vi "Compress with 7Zip.vi"(8 "error in (no error)":errorcluster, 9 "Compressed File Type":string(combo)="7z", 10 "7z File to compress into":path=path "D:/Ab-initio/VASP Calcs/1D_Dislocations/Batch04_20130519/1_DOS.7z", 11 "Folder or file to compress":path=path "D:/Ab-initio/VASP Calcs/1D_Dislocations/Batch04_20130519/1_DOS") -> (0 "error out":errorcluster)   [LabVIEW 2010]
panel:
  out "concatenated string":string="\"C:\\Program Files\\7-Zip\\7za.exe\" a -t7z \"D:\\Ab-initio\\VASP Calcs\\1D_Dislocations\\Batch04_20130519\\1_DOS.7Z\" \"D:\\Ab-initio\\VASP Calcs\\1D_Dislocations\\Batch04_20130519\\1_DOS\""
  in  "7za.exe path":path=path "C:/Program Files/7-Zip/7za.exe"
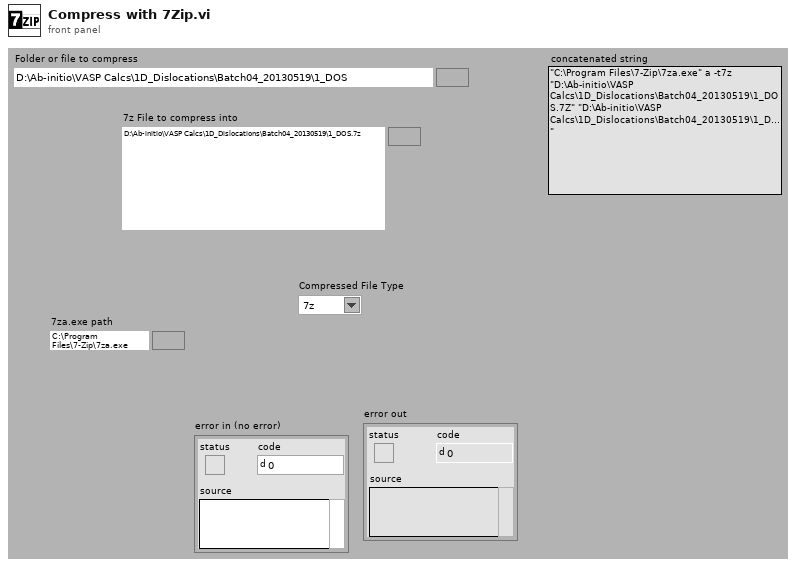
[diagram p1: front panel]
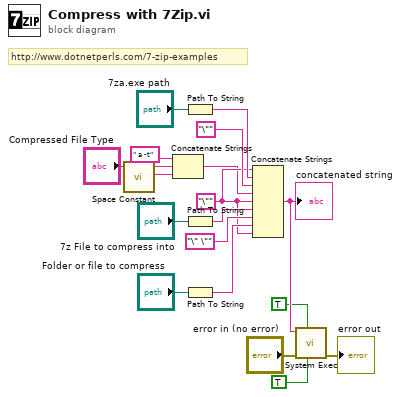
[diagram p0: block diagram]
diagram:
  w11 = "\"" ("string")
  # "http://www.dotnetperls.com/7-zip-examples"
  n1 = call <vilib>:"Space Constant.vi"() -> ("String"=w6:string)
  n2 = Concatenate Strings(" a -t" ("string"), "Compressed File Type", w6) -> (w5:string)
  n3 = Path To String(path="7za.exe path") -> (string=w17:string)
  n4 = Path To String(path="7z File to compress into") -> (string=w16:string)
  n5 = Path To String(path="Folder or file to compress") -> (string=w13:string)
  n6 = Concatenate Strings(w11, w17, "\"" ("string"), w5, w11, w16, "\" \"" ("string"), w13, w11) -> (w10:string)
  "concatenated string" <- w10
  n7 = call <vilib>:"System Exec.vi"("run minimized? (F)"=TRUE, "wait until completion? (T)"=TRUE, "error in (no error)"="error in (no error)", "command line"=w10) -> ("error out"=→"error out":errorcluster)  [unwired: 4 in, 3 out]
